vi "fish out reply.vi"(2 "predetermined prompt without $":string, 3 "error in":errorcluster, 4 "original command":string="whoami", 5 "total output":string="whoami\r\ngit\r\ngit@hosman7dt3500-ubuntu:~$ \r\ngit@hosman7dt3500-ubuntu:~$ ") -> (0 "error out":errorcluster, 1 "final match":string)   [LabVIEW 2016, in "labssh_thijs.lvlib"]
uses:
  <vilib>/regexp/Match Regular Expression.xnode
  labssh_thijs.lvlib
panel:
  out "after match 3":string
  out "whole match 3":string
  out "after match 2":string
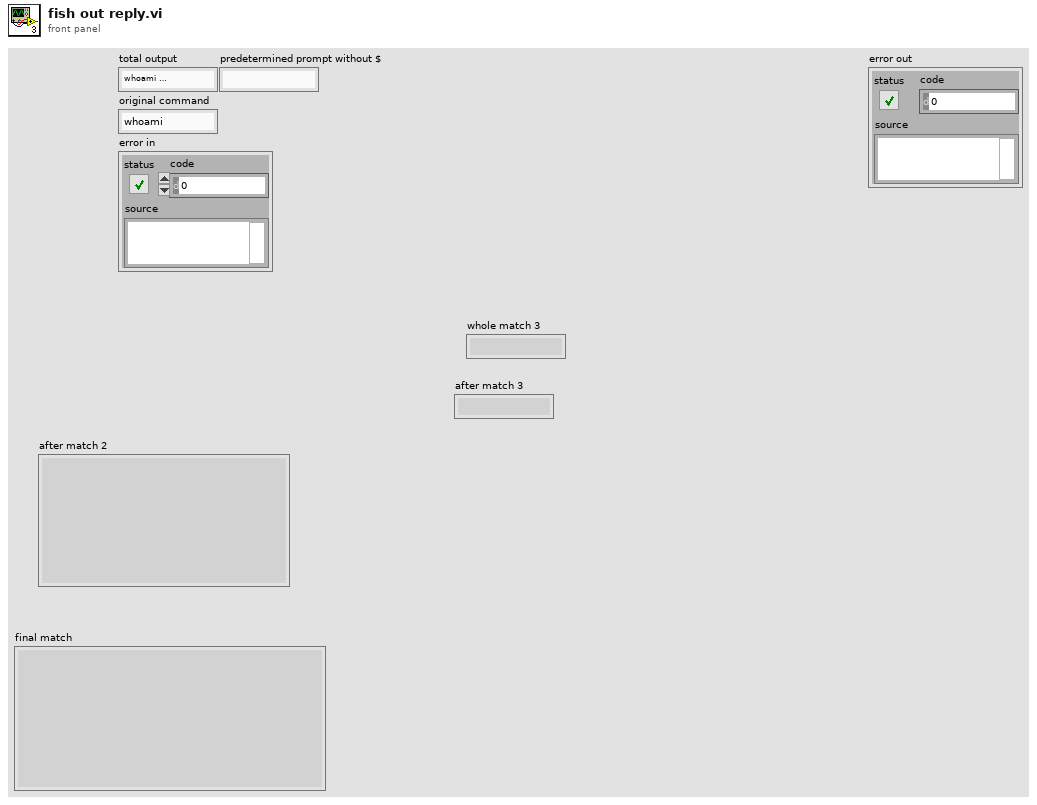
[diagram p1: front panel]
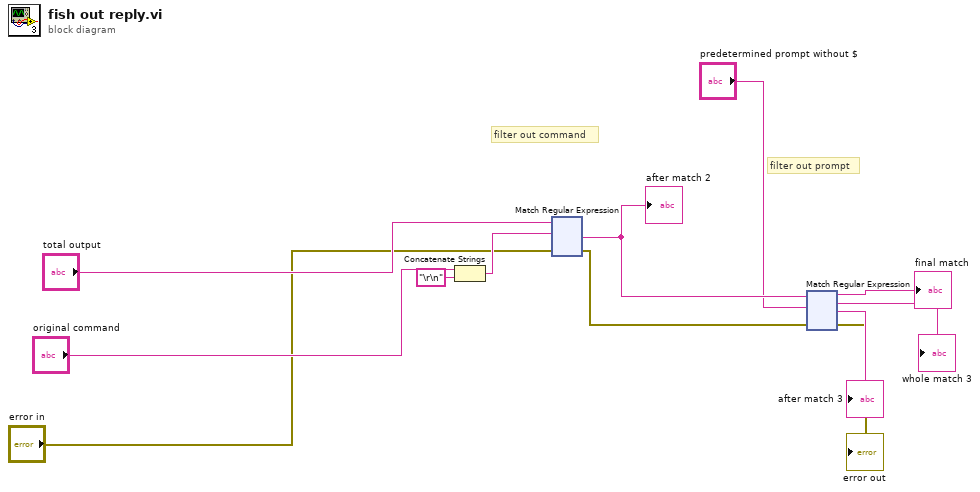
[diagram p0: block diagram]
diagram:
  # "filter out prompt"
  # "filter out command"
  n1 = Concatenate Strings("original command", "\r\n" ("string")) -> (w9:string)
  n2 = xnode "Match Regular Expression"("input string"="total output", "regular expression"=w9, "error in"="error in") -> ("after match"=w8:string, "error out"=w3:errorcluster)  [unwired: 3 in, 3 out]
  "after match 2" <- w8
  n3 = xnode "Match Regular Expression"("input string"=w8, "regular expression"="predetermined prompt without $", "error in"=w3) -> ("before match"=→"final match":string, "whole match"=→"whole match 3":string, "after match"=→"after match 3":string, "error out"=→"error out":errorcluster)  [unwired: 3 in, 1 out]
